vi "post_vi_data.vi"() -> ()   [LabVIEW 2019]
uses:
  <vilib>/httpClient/POSTBuffer.vi
  <vilib>/httpClient/LabVIEWHTTPClient.lvlib
panel:
  out "headers":string
  out "body":string
  in  "url":string
  out "Number of Files":i32
  in  "Target Path":path
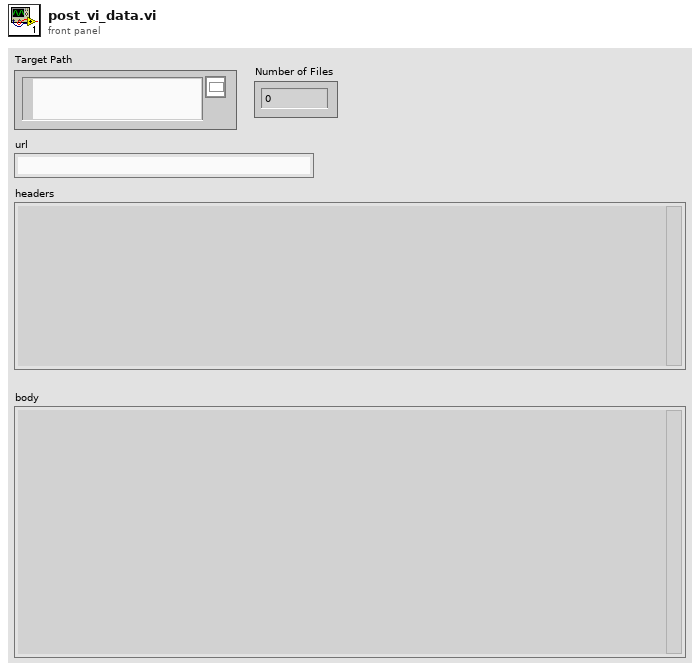
[diagram p1: front panel]
types:
  T1 = typedef "LabVIEWHTTPClient.lvlib/ClientHandle.ctl" = refnum<k1>
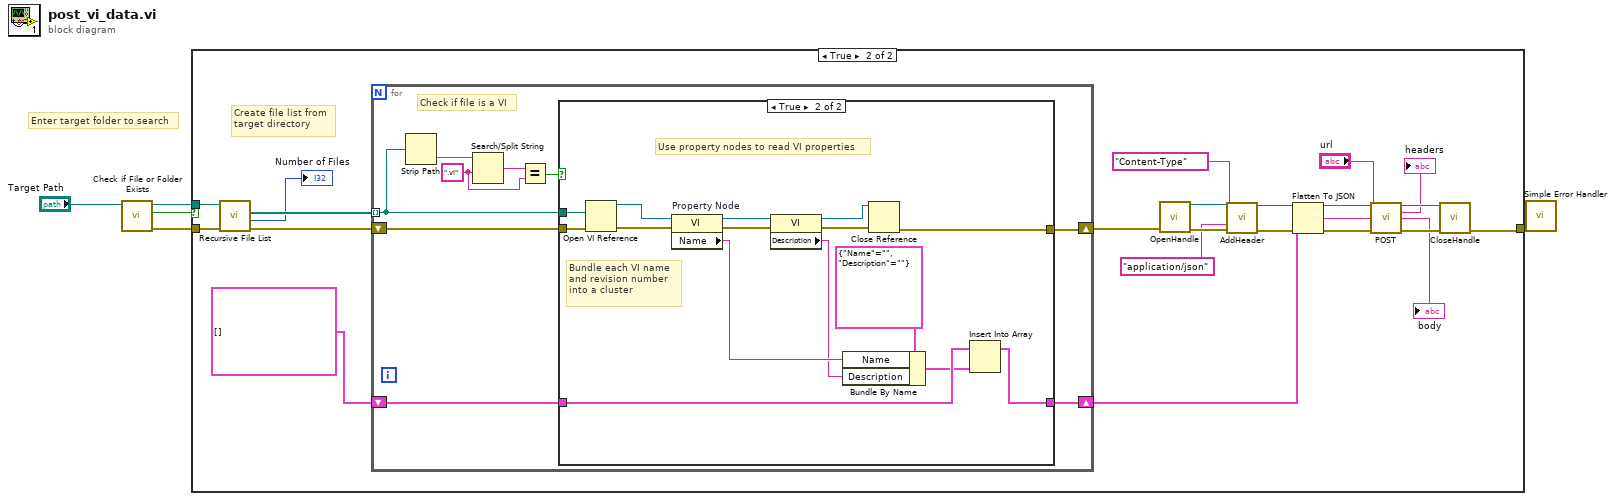
[diagram p0: block diagram]
diagram:
  # "Enter target folder to search"
  n1 = call <vilib>:"Check if File or Folder Exists.vi"("path"="Target Path") -> ("error out"=w2:errorcluster, "file or folder exists?"=w5:bool, "dup path"=w4:path)  [unwired: 8 in]
  n2 = case shown="True" w5 {
    tunnel: w4 -> [_ w27]
    tunnel: w2 -> [w6 w28]
    tunnel: [w6 w19] -> w1
    frame False {
    }
    frame True {
      # "Create file list from\ntarget directory"
      n3 = call <vilib>:"Recursive File List.vi"("error in (no error)"=w28, "Folder Path"=w27) -> ("error out"=w24:errorcluster, "Number of Files"=→"Number of Files":i32, "All Files in Dir"=w26:path[])  [unwired: 5 in, 2 out]
      n4 = for {
        tunnel: w26 -> [w32] mode=indexing
        shift-right: [w31] -> w22
        shift-left: w24 -> [w33]
        shift-right: [w29] -> w12
        shift-left: cluster{"Name":string, "Description":string}[] [] -> [w30]
        w35 = ".vi" ("search string/char (-)")
        # "Check if file is a VI"
        n5 = Strip Path(path=w32) -> (name=w37:string)  [unwired: 1 out]
        n6 = Search/Split String(string=w37, search string/char (-)=w35) -> (match + rest of string=w36:string)  [unwired: 1 in, 2 out]
        n7 = Equal?(x=w36, y=w35) -> (x = y?=w34:bool)
        n8 = case shown="True" w34 {
          tunnel: w33 -> [w39 w54]
          tunnel: w32 -> [_ w53]
          tunnel: [w39 w50] -> w31
          tunnel: w30 -> [w38 w42]
          tunnel: [w38 w40] -> w29
          frame False {
          }
          frame True {
            # "Use property nodes to read VI properties"
            # "Bundle each VI name\nand revision number\ninto a cluster"
            n9 = Open VI Reference(vi path=w53, error in (no error)=w54) -> (vi reference=w52:refnum<vi>, error out=w51:errorcluster)  [unwired: 4 in]
            n10 = property on="Property Node" class="VI"(reference=w52, error in=w51) -> (reference out=w49:refnum<vi>, error out=w48:errorcluster, "Name"=w45:string)
            n11 = property class="VI"(reference=w49, error in=w48) -> (reference out=w46:refnum<vi>, error out=w47:errorcluster, "Description"=w44:string)
            n12 = Bundle By Name(cluster=cluster{"Name":string, "Description":string} {"Name"="", "Description"=""}, "Name"=w45, "Description"=w44) -> (w41:cluster{"Name":string, "Description":string})
            n13 = Close Reference(reference=w46, error in (no error)=w47) -> (error out=w50:errorcluster)
            n14 = Insert Into Array(array=w42, new element=w41) -> (w40:cluster{"Name":string, "Description":string}[])  [unwired: 1 in]
          }
        }
      }
      n15 = call <vilib>:"OpenHandle.vi"("error in (no error)"=w22) -> ("client handle out"=w18:T1, "error out"=w21:errorcluster)  [unwired: 13 in]
      n16 = call <vilib>:"AddHeader.vi"("client handle"=w18, "header"="Content-Type", "value"="application/json", "error in (no error)"=w21) -> ("client handle out"=w17:T1, "error out"=w10:errorcluster)  [unwired: 10 in]
      n17 = Flatten To JSON(anything=w12, error in (no error)=w10) -> (JSON string=w11:string, 11:w9:errorcluster)  [unwired: 1 in]
      n18 = call-poly <vilib>:"POST.vi"("client handle"=w17, "url"="url", "buffer"=w11, "error in (no error)"=w9) -> ("client handle out"=w16:T1, "headers"=→"headers":string, "body"=→"body":string, "error out"=w20:errorcluster)  [unwired: 8 in]
      n19 = call <vilib>:"CloseHandle.vi"("client handle"=w16, "error in (no error)"=w20) -> ("error out"=w19:errorcluster)  [unwired: 13 in]
    }
  }
  n20 = call <vilib>:"Simple Error Handler.vi"("error in (no error)"=w1) -> ()  [unwired: 4 in, 5 out]
